vi "MainRT.vi"() -> ()   [LabVIEW 2017]
uses:
  Projekt-RubikLibrary/RubikLibrary.lvlib
panel:
  out "Succes?":bool
  in  "Exit":bool
  in  "Start":bool
  # "Test: Rubik's Cube Startup"
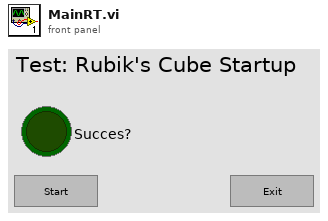
[diagram p1: front panel]
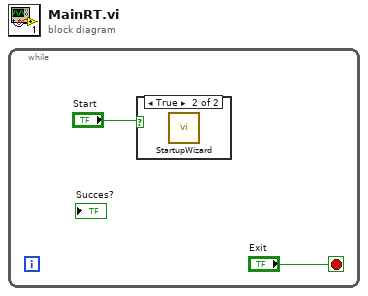
[diagram p0: block diagram]
diagram:
  n1 = while {
    stop <- "Exit" stop-if-true
    n2 = case shown="True" "Start" {
      frame False {
      }
      frame True {
        n3 = call "StartupWizard.vi"() -> ()  [unwired: 1 in, 1 out]
      }
    }
  }
